vi "Wrapper.vi"(8 "error in":errorcluster, 10 "Voltage":dbl, 11 "gController in":refnum<class "gController.lvclass">) -> (0 "error out":errorcluster, 3 "Actor out":refnum<class "Actor.lvclass">)   [LabVIEW 2017, in "Controller.lvlib" / "Update Fan Voltage MSG.lvclass"]
uses:
  Update Fan Voltage MSG.lvclass
  gController.lvclass
  C:/Program Files (x86)/National Instruments/LabVIEW 2017/vi.lib/ActorFramework/Actor/Actor.lvclass
  <vilib>/ActorFramework/Actor/Actor.lvclass
  <vilib>/Utility/error.llb/Error Cluster From Error Code.vi
  <vilib>/rvi/errors/niLvFpgaAdjustHostInterfaceError.vi
  <vilib>/rvi/interface/nirviReadWriteControl/nirviReadWriteControl.xnode
  FPGA Ref.ctl
  FPGA Bitfiles/server.lvbitx
  NiFpgaLv.dll
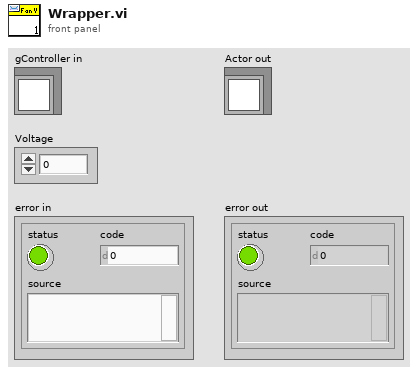
[diagram p1: front panel]
types:
  T1 = typedef "FPGA Ref.ctl" = refnum<k20>
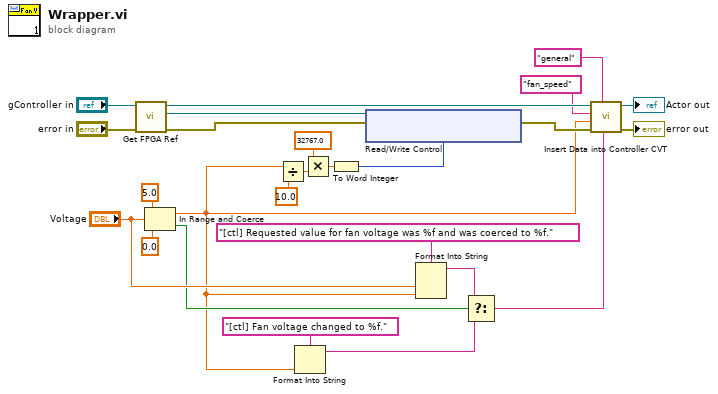
[diagram p0: block diagram]
diagram:
  n1 = call "Get FPGA Ref.vi"("error in (no error)"="error in", "Actor In"="gController in") -> ("error out"=w24:errorcluster, "FPGA Ref"=w23:T1, "Actor Out"=w25:refnum<class "Actor.lvclass">)  [unwired: 7 in]
  n2 = In Range and Coerce(upper limit=5.0, x="Voltage", lower limit=0.0) -> (coerced(x)=w5:dbl, In Range?=w12:bool)
  n3 = Divide(x=w5, y=10.0) -> (x/y=w3:dbl)
  n4 = Format Into String(format string="[ctl] Fan voltage changed to %f.", w5) -> (resulting string=w17:string)  [unwired: 2 in, 1 out]
  n5 = Multiply(x=32767.0 ("n"), y=w3) -> (x*y=w1:dbl)
  n6 = To Word Integer(number=w1) -> (16bit integer=w8:i16)
  n7 = xnode "Read/Write Control"("FPGA VI Reference In"=w23, "error in"=w24, "Fan Voltage"=w8) -> ("error out"=w19:errorcluster)  [unwired: 1 out]
  n8 = Format Into String(format string="[ctl] Requested value for fan voltage was %f and was coerced to %f.", "Voltage", w5) -> (resulting string=w15:string)  [unwired: 2 in, 1 out]
  n9 = Select(t=w15, s=w12, f=w17) -> (s? t:f=w18:string)
  n10 = call "Insert Data into Controller CVT.vi"("Update MSG"=w18, "Group"="general", "error in"=w19, "Data"=w5, "tag"="fan_speed", "Actor in"=w25) -> ("error out"=→"error out":errorcluster, "Actor Out"=→"Actor out":refnum<class "Actor.lvclass">)  [unwired: 4 in]
